vi "MGI Wrap Word to Pixel Width.vi"(6 "Allowed Width":i16, 8 "Word":string, 9 "Word Width(pixels)":i16, 10 "Font":T1={"Font Name:"="", "Size"=12, "Strikeout?"=FALSE, "Italic?"=FALSE, "Underline?"=FALSE, "Outline?"=FALSE, "Shadow?"=FALSE, "Bold?"=FALSE}, 11 "Start String":string) -> (3 "String Out":string, 4 "Width Used":i16)   [LabVIEW 2016]
doc: "Perform a word wrap operation on a single word which may need to be broken into parts. Start string must be empty or end in a line feed.\n\nAuthored by David A. Moore\nsupport@mooregoodideas.com\nwww.mooregoodideas.com\n\nCopyright (c) 2010, Moore Good Ideas, Inc.\n\nAll rights reserved.\n\nRedistribution and use in source and binary forms, with or without modification, are permitted provided that the following conditions are met:\n\n * Redistributions of source code must retain the above copyright notice, this list of conditions and the following disclaimer.\n * Redistributions in binary form must reproduce the above copyright notice, this list of conditions and the following disclaimer in the documentation and/or other materials provided with the distribution.\n * Neither the name of Moore Good Ideas, Inc. nor the names of its contributors may be used to endorse or promote products derived from this software without specific prior written permission.\n\nTHIS SOFTWARE IS PROVIDED BY THE COPYRIGHT HOLDERS AND CONTRIBUTORS \"AS IS\" AND ANY EXPRESS OR IMPLIED WARRANTIES, INCLUDING, BUT NOT LIMITED TO, THE IMPLIED WARRANTIES OF MERCHANTABILITY AND FITNESS FOR A PARTICULAR PURPOSE ARE DISCLAIMED. IN NO EVENT SHALL THE COPYRIGHT OWNER OR CONTRIBUTORS BE LIABLE FOR ANY DIRECT, INDIRECT, INCIDENTAL, SPECIAL, EXEMPLARY, OR CONSEQUENTIAL DAMAGES (INCLUDING, BUT NOT LIMITED TO, PROCUREMENT OF SUBSTITUTE GOODS OR SERVICES; LOSS OF USE, DATA, OR PROFITS; OR BUSINESS INTERRUPTION) HOWEVER CAUSED AND ON ANY THEORY OF LIABILITY, WHETHER IN CONTRACT, STRICT LIABILITY, OR TORT (INCLUDING NEGLIGENCE OR OTHERWISE) ARISING IN ANY WAY OUT OF THE USE OF THIS SOFTWARE, EVEN IF ADVISED OF THE POSSIBILITY OF SUCH DAMAGE."
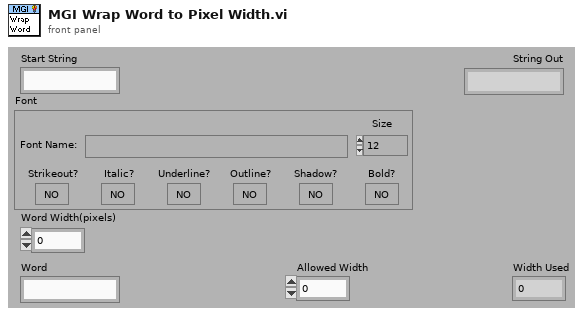
[diagram p1: front panel]
types:
  T1 = cluster{"Font Name:":string, "Size":i16, "Strikeout?":bool, "Italic?":bool, "Underline?":bool, "Outline?":bool, "Shadow?":bool, "Bold?":bool}
  T2 = enum16{"User-specified Font", "Application Font", "System Font", "Dialog Font"}
  T3 = cluster{"left":i16, "top":i16, "right":i16, "bottom":i16}
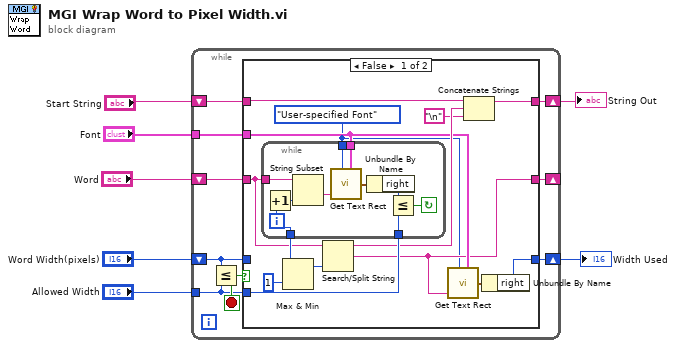
[diagram p0: block diagram]
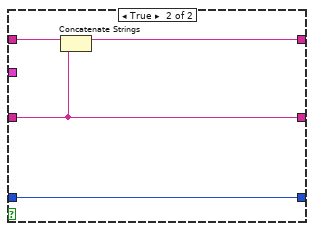
[diagram p2: hidden frame]
diagram:
  n1 = while {
    tunnel: "Font" -> [w8]
    tunnel: "Allowed Width" -> [w9]
    shift-left: "Word Width(pixels)" -> [w15]
    shift-right: [w14] -> w3
    shift-left: "Word" -> [w13]
    shift-right: [w10] -> _
    shift-left: "Start String" -> [w12]
    shift-right: [w11] -> w1
    stop <- w16 stop-if-true
    n2 = Less Or Equal?(x=w15, y=w9) -> (x <= y?=w16:bool)
    n3 = case shown="False" w16 {
      tunnel: w15 -> [_ w44]
      tunnel: [w17 w44] -> w14
      tunnel: w13 -> [w27 w41]
      tunnel: w12 -> [w24 w43]
      tunnel: [w25 w42] -> w11
      tunnel: [w20 w41] -> w10
      tunnel: w9 -> [w30 _]
      tunnel: w8 -> [w21 _]
      frame False {
        w19 = T2."User-specified Font" ("desired font(application)")
        n4 = while {
          tunnel: w19 -> [w31]
          tunnel: [w32] -> w29
          tunnel: w30 -> [w35]
          tunnel: w21 -> [w38]
          tunnel: w27 -> [w40]
          i -> [w32]
          stop <- w34 continue-if-true
          n5 = Increment(x=w32) -> (x+1=w33:i32)
          n6 = String Subset(string=w40, length (rest)=w33) -> (substring=w39:string)  [unwired: 1 in]
          n7 = call <vilib>:"Get Text Rect.vi"("desired font(Application)"=w31, "text"=w39, "[user-specified font]"=w38) -> ("rect"=w37:T3)  [unwired: 6 in]
          n8 = Unbundle By Name(w37) -> ("right"=w36:i16)
          n9 = Less Or Equal?(x=w36, y=w35) -> (x <= y?=w34:bool)
        }
        n10 = Max & Min(x=w29, y=1) -> (max(x,y)=w26:i32)  [unwired: 1 out]
        n11 = Search/Split String(string=w27, offset (0)=w26) -> (substring before match=w23:string, match + rest of string=w20:string)  [unwired: 1 in, 1 out]
        n12 = call <vilib>:"Get Text Rect.vi"("desired font(Application)"=w19, "text"=w20, "[user-specified font]"=w21) -> ("rect"=w18:T3)  [unwired: 6 in]
        n13 = Concatenate Strings(w24, w23, "\n") -> (w25:string)
        n14 = Unbundle By Name(w18) -> ("right"=w17:i16)
      }
      frame True {
        n15 = Concatenate Strings(w43, w41) -> (w42:string)
      }
    }
  }
  "Width Used" <- w3
  "String Out" <- w1
